vi "configure.vi"(8 "error in (no error)":errorcluster, 11 "ILCSim1 in":refnum<class "ILCSim1.lvclass">) -> (0 "error out":errorcluster, 3 "ILCSim1 out":refnum<class "ILCSim1.lvclass">)   [LabVIEW 2013, in "ILCSim1.lvclass"]
uses:
  <userlib>/Common/Simulators/ILCSim1/ILCSim1.lvclass
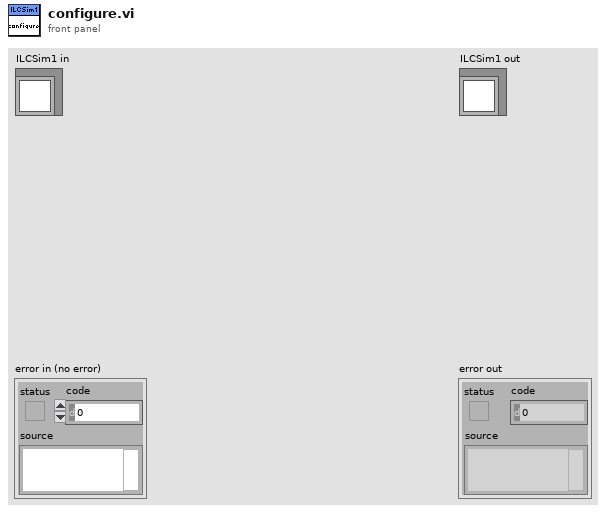
[diagram p1: front panel]
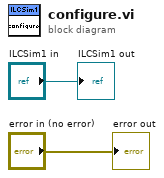
[diagram p0: block diagram]
diagram:
  "error out" <- "error in (no error)"
  "ILCSim1 out" <- "ILCSim1 in"
